vi "SV Get By Measurement Type (tach) (1 Ch).vi"(0 "scaled signals [EU]":waveform(dbl)[](array[waveform])) -> (4 "scaled signals with tachometer channel deleted":waveform(dbl)[](array[waveform]), 6 "found?":bool, 8 "tachometer channel":waveform(dbl), 10 "threshold":dbl, 12 "maximum order":i32, 13 "rotation direction":u16(ring) items=["CCW", "CW"], 14 "slope":u16(ring) items=["Rising", "Falling"], 15 "pulses per rev":i32)   [LabVIEW 2017]
doc: "Separates data from an array of waveforms based on the type of measurement selected. This VI requires that waveform attributes such as NI_UnitDescription are added by NI DAQmx."
uses:
  <vilib>/addons/_NISVFA/_Shared subVIs/Controls/SV Channel Properties.ctl
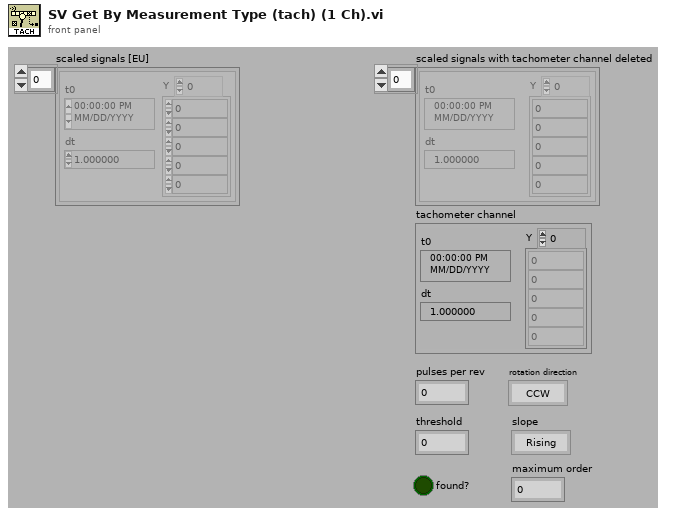
[diagram p1: front panel]
types:
  T1 = typedef "SV Channel Properties.ctl" = u16
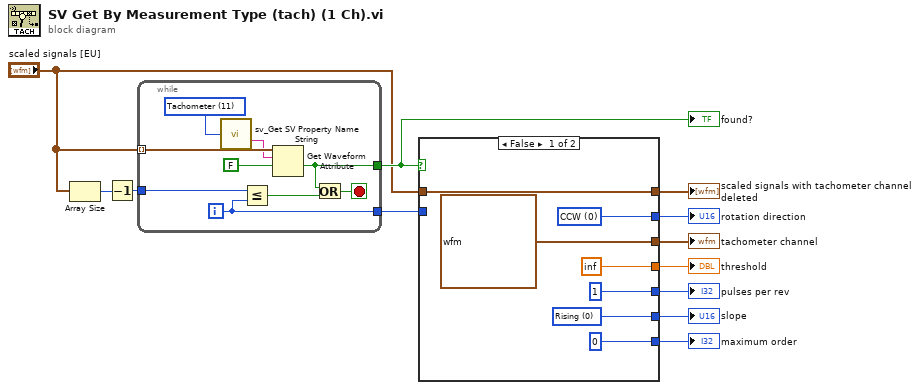
[diagram p0: block diagram]
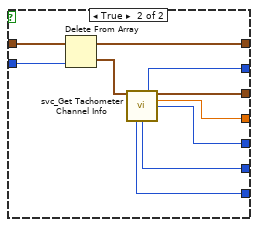
[diagram p2: hidden frame]
diagram:
  n1 = Array Size(array="scaled signals [EU]") -> (size(s)=w12:i32)
  n2 = Decrement(x=w12) -> (x-1=w11:i32)
  n3 = while {
    tunnel: "scaled signals [EU]" -> [w21] mode=indexing
    tunnel: w11 -> [w20]
    tunnel: [w17] -> w10
    tunnel: [w16] -> w8
    i -> [w16]
    stop <- w19 stop-if-true
    w13 = T1 11 items=["Engineering units", "Custom unit label", "Weighting filter", "Pregain", "Octave standard", "Octave bandwidth", "Octave low band", "Octave high band", "Spectrum skewed", "Samples / revolution", "Order", "Tachometer", "Pulses Per Revolution", "Rotation Direction", "Probe Angle", "Pair", "Channel Alias", "Tachometer Threshold", "Tachometer Slope", "Max Order", "Sensor Location", "Sensor Orientation"] ("property")
    n4 = call <vilib>:"sv_Get SV Property Name String.vi"("property"=w13) -> ("WDT attribute name"=w14:string)  [unwired: 13 in, 1 out]
    n5 = Less Or Equal?(x=w20, y=w16) -> (x <= y?=w18:bool)
    n6 = Get Waveform Attribute(5:FALSE, 6:w14, 7:w21) -> (1:w17:bool)  [unwired: 1 in, 3 out]
    n7 = Or(x=w17, y=w18) -> (x .or. y?=w19:bool)
  }
  "found?" <- w10
  n8 = case shown="False" w10 {
    tunnel: "scaled signals [EU]" -> [w28 w38]
    tunnel: w8 -> [_ w37]
    tunnel: [w28 w36] -> w7
    tunnel: [waveform(dbl) {"t0"=timestamp(0 s since 1904-01-01), "dt"=1.0, "Y"=[]} ("Waveform") w34] -> w6
    tunnel: [1 w33] -> w5
    tunnel: [w22 w29] -> w4
    tunnel: [inf w32] -> w3
    tunnel: [w23 w30] -> w1
    tunnel: [0 w31] -> w2
    frame False {
      w22 = u16 0 items=["CCW", "CW"] ("rotation direction")
      w23 = u16 0 items=["Rising", "Falling"] ("slope (Rising)")
    }
    frame True {
      n9 = Delete From Array(array=w38, index=w37) -> (deleted portion=w35:waveform(dbl), array with subset deleted=w36:waveform(dbl)[])  [unwired: 1 in]
      n10 = call <vilib>:"svc_Get Tachometer Channel Info.vi"("Tachometer Channel in"=w35) -> ("rotation direction"=w29:u16, "Tachometer Channel out"=w34:waveform(dbl), "Threshold"=w32:dbl, "Pulses Per Rev"=w33:i32, "Max Order"=w31:i32, "Slope"=w30:u16)  [unwired: 9 in]
    }
  }
  "tachometer channel" <- w6
  "scaled signals with tachometer channel deleted" <- w7
  "pulses per rev" <- w5
  "rotation direction" <- w4
  "threshold" <- w3
  "slope" <- w1
  "maximum order" <- w2
